vi "Calc Axis Attributes_modded.vi"(0 "rect":T7, 1 "desired font(Application)":T5(ring)=enum."Application Font", 2 "xy axis":T1={"x minimum"=0.0, "x maximum"=0.0, "x log?"=FALSE, "x precision"=1, "x format"=enum."Decimal", "y minimum"=0.0, "y maximum"=0.0, "y log?"=FALSE, "y precision"=1, "y format"=enum."Decimal"} {"x minimum" format="%.2f"; "x maximum" format="%.2f"; "y minimum" format="%.2f"; "y maximum" format="%.2f"}, 3 "grid cosmetics":T2={"line color"=39168, "text color"=65280, "tick length"=3, "crossing axes"=FALSE, "visible grid?"=TRUE}, 5 "[user-specified font]":T6) -> (7 "x axis attributes":T4 {"value 2" format="%.2f"; "value 1" format="%.2f"}, 9 "y axis attributes":T4 {"value 2" format="%.2f"; "value 1" format="%.2f"})   [LabVIEW 2018]
uses:
  fmt_prec_modded.ctl
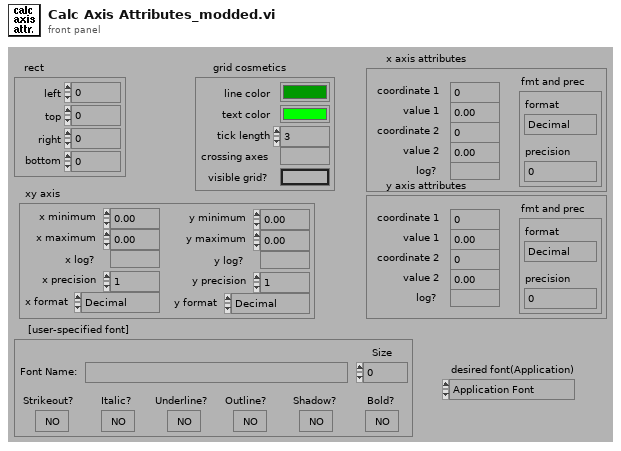
[diagram p1: front panel]
types:
  T1 = cluster{"x minimum":dbl, "x maximum":dbl, "x log?":bool, "x precision":u8, "x format":enum8{"Decimal", "Scientific", "Engineering", "Binary", "Octal", "Hex", "Timestamp"}, "y minimum":dbl, "y maximum":dbl, "y log?":bool, "y precision":u8, "y format":enum8{"Decimal", "Scientific", "Engineering", "Binary", "Octal", "Hex", "Timestamp"}}
  T2 = cluster{"line color":u32, "text color":u32, "tick length":i16, "crossing axes":bool, "visible grid?":bool}
  T3 = typedef "fmt_prec_modded.ctl" = cluster{"format":enum8{"Decimal", "Scientific", "Engineering", "Binary", "Octal", "Hex", "Timestamp"}, "precision":u8}
  T4 = cluster{"coordinate 1":i16, "value 1":dbl, "coordinate 2":i16, "value 2":dbl, "log?":bool, "fmt and prec":T3}
  T5 = enum16{"User-specified Font", "Application Font", "System Font", "Dialog Font"}
  T6 = cluster{"Font Name:":string, "Size":i16, "Strikeout?":bool, "Italic?":bool, "Underline?":bool, "Outline?":bool, "Shadow?":bool, "Bold?":bool}
  T7 = cluster{"left":i16, "top":i16, "right":i16, "bottom":i16}
  T8 = enum8{"Decimal", "Scientific", "Engineering", "Binary", "Octal", "Hex", "Timestamp"}
  T9 = cluster{"x format":enum8{"Decimal", "Scientific", "Engineering", "Binary", "Octal", "Hex", "Timestamp"}, "x precision":u8}
  T10 = cluster{"y format":enum8{"Decimal", "Scientific", "Engineering", "Binary", "Octal", "Hex", "Timestamp"}, "y precision":u8}
  T11 = cluster{"left":i16, "x minimum":dbl, "right":i16, "x maximum":dbl, "x log?":bool, cluster{"x format":enum8{"Decimal", "Scientific", "Engineering", "Binary", "Octal", "Hex", "Timestamp"}, "x precision":u8}}
  T12 = cluster{"bottom":i16, "y minimum":dbl, "top":i16, "y maximum":dbl, "y log?":bool, cluster{"y format":enum8{"Decimal", "Scientific", "Engineering", "Binary", "Octal", "Hex", "Timestamp"}, "y precision":u8}}
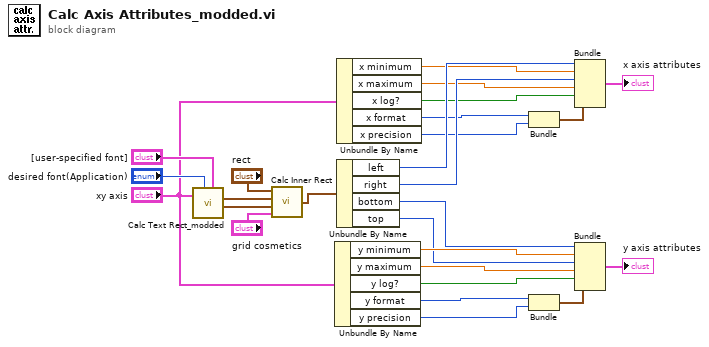
[diagram p0: block diagram]
diagram:
  n1 = call "Calc Text Rect_modded.vi"("xy axis"="xy axis", "desired font(Application)"="desired font(Application)", "[user-specified font]"="[user-specified font]") -> ("y rect"=w14:T7, "x rect"=w15:T7)  [unwired: 3 in]
  n2 = call <vilib>:"Calc Inner Rect.vi"("grid cosmetics"="grid cosmetics", "y text rect"=w14, "x text rect"=w15, "graph rect"="rect") -> ("inner rect"=w10:T7)
  n3 = Unbundle By Name("xy axis") -> ("y minimum"=w22:dbl, "y maximum"=w21:dbl, "y log?"=w13:bool, "y format"=w5:T8, "y precision"=w4:u8)
  n4 = Unbundle By Name("xy axis") -> ("x minimum"=w25:dbl, "x maximum"=w23:dbl, "x log?"=w12:bool, "x format"=w8:T8, "x precision"=w7:u8)
  n5 = Unbundle By Name(w10) -> ("left"=w26:i16, "right"=w24:i16, "bottom"=w2:i16, "top"=w1:i16)
  n6 = Bundle("x format"=w8, "x precision"=w7) -> (w6:T9)  [unwired: 1 in]
  n7 = Bundle("y format"=w5, "y precision"=w4) -> (w3:T10)  [unwired: 1 in]
  n8 = Bundle("left"=w26, "x minimum"=w25, "right"=w24, "x maximum"=w23, "x log?"=w12, w6) -> (→"x axis attributes":T11)  [unwired: 1 in]
  n9 = Bundle("bottom"=w2, "y minimum"=w22, "top"=w1, "y maximum"=w21, "y log?"=w13, w3) -> (→"y axis attributes":T12)  [unwired: 1 in]
